vi "Configure Heads.vi"(6 "Operation (0: Add)":i32(ring) items=["Add", "Delete", "Select"], 7 "Head Position (0)":i32, 8 "error in (no error)":errorcluster, 9 "Head Model (\"\")":string="\"\"", 10 "Channel (1: Channel 1)":i32(ring)=1 items=["Channel 1"=1, "Channel 2"=2, "Channel 3"=3, "Channel 4"=4], 11 "VISA resource name":refnum<visa-resource-name>) -> (0 "error out":errorcluster, 3 "VISA resource name out":refnum<visa-resource-name>)   [LabVIEW 2020, in "Agilent 90000 Series.lvlib"]
doc: "Configure settings for probe heads."
uses:
  Agilent 90000 Series.lvlib
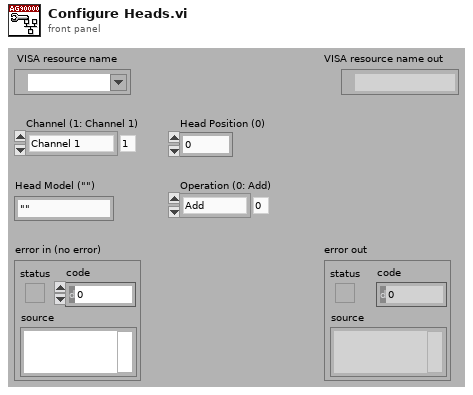
[diagram p1: front panel]
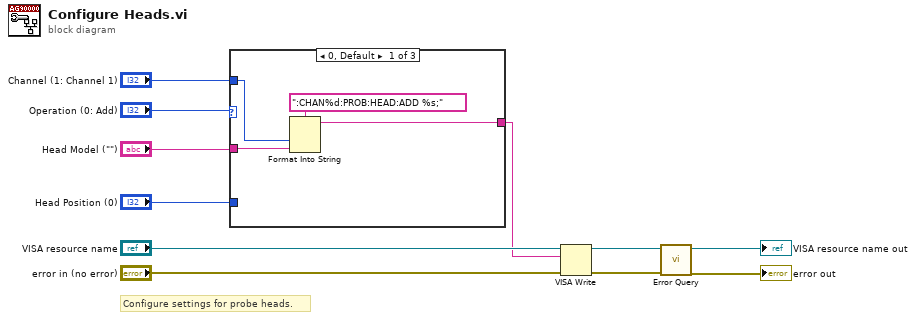
[diagram p0: block diagram]
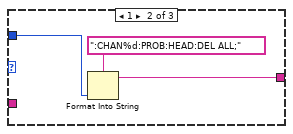
[diagram p2: hidden frame]
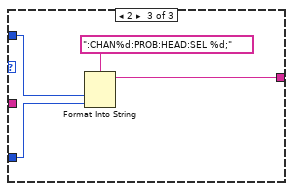
[diagram p3: hidden frame]
diagram:
  # "Configure settings for probe heads."
  n1 = case shown="0, Default" "Operation (0: Add)" {
    tunnel: "Channel (1: Channel 1)" -> [w14 w18 w20]
    tunnel: "Head Model (\"\")" -> [w13 _ _]
    tunnel: [w12 w16 w22] -> w1
    tunnel: "Head Position (0)" -> [_ _ w19]
    frame 0, Default {
      n2 = Format Into String(format string=":CHAN%d:PROB:HEAD:ADD %s;", w14, w13) -> (resulting string=w12:string)  [unwired: 2 in, 1 out]
    }
    frame 1 {
      n3 = Format Into String(format string=":CHAN%d:PROB:HEAD:DEL ALL;", w18) -> (resulting string=w16:string)  [unwired: 2 in, 1 out]
    }
    frame 2 {
      n4 = Format Into String(format string=":CHAN%d:PROB:HEAD:SEL %d;", w20, w19) -> (resulting string=w22:string)  [unwired: 2 in, 1 out]
    }
  }
  n5 = VISA Write(VISA resource name="VISA resource name", write buffer=w1, error in (no error)="error in (no error)") -> (VISA resource name out=w9:refnum<visa-resource-name>, error out=w8:errorcluster)  [unwired: 1 out]
  n6 = call "Error Query.vi"("error in (no error)"=w8, "VISA resource name"=w9) -> ("error out"=→"error out":errorcluster, "VISA resource name out"=→"VISA resource name out":refnum<visa-resource-name>)  [unwired: 8 out]
